vi "Create All Message Queues.vi"(8 "error in (no error)":cluster{"状态":bool, "代码":i32, "源":string} caption="错误输入（无错误）") -> (0 "error out":cluster{"状态":bool, "代码":i32, "源":string} caption="错误输出", 3 "消息队列输出":T1)   [LabVIEW 2014, in "Message Queue.lvlib"]
doc: "本VI用于创建应用程序所需的所有消息队列。如应用程序需要两个以上消息队列，可右键单击上面的“消息队列”常量并选择“打开自定义类型”，将新的消息队列添加至该自定义类型，然后通过本VI进行初始化。"
uses:
  Message Queue.lvlib
  All Message Queues.ctl
  Message Cluster.ctl
  Enqueue Message (Single).vi
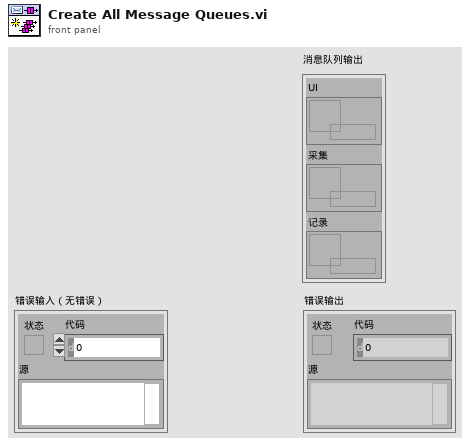
[diagram p1: front panel]
types:
  T1 = typedef "Message Queue.lvlib/All Message Queues.ctl" = cluster{"UI":refnum<queue>, "采集":refnum<queue>, "记录":refnum<queue>}
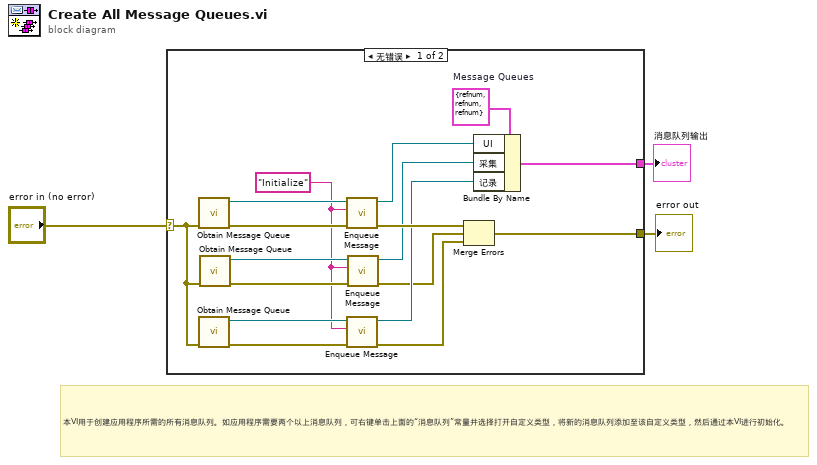
[diagram p0: block diagram]
diagram:
  # "本VI用于创建应用程序所需的所有消息队列。如应用程序需要两个以上消息队列，可右键单击上面的“消息队列”常量并选择打开自定义类型，将新的消息队列添加至该自定义类型，然后通过本VI进行初始化。"
  n1 = case shown="无错误" "error in (no error)" {
    selector: "error in (no error)" -> [w11 w21]
    tunnel: [w6 w21] -> w3
    tunnel: [w18 _] -> w2
    frame No Error {
      w10 = "Initialize" ("Message")
      w19 = T1 {"UI"=refnum, "采集"=refnum, "记录"=refnum}  # Message Queues
      n2 = call "Obtain Message Queue.vi"("error in (no error)"=w11) -> ("error out"=w17:cluster{"状态":bool, "代码":i32, "源":string}, "消息队列"=w16:refnum<queue>)  [unwired: 9 in]
      n3 = call "Obtain Message Queue.vi"("error in (no error)"=w11) -> ("error out"=w13:cluster{"状态":bool, "代码":i32, "源":string}, "消息队列"=w12:refnum<queue>)  [unwired: 9 in]
      n4 = call "Obtain Message Queue.vi"("error in (no error)"=w11) -> ("error out"=w14:cluster{"状态":bool, "代码":i32, "源":string}, "消息队列"=w15:refnum<queue>)  [unwired: 9 in]
      n5 = call-poly "Enqueue Message.vi"("error in (no error)"=w17, "消息"=w10, "消息队列"=w16) -> ("error out"=w20:cluster{"状态":bool, "代码":i32, "源":string}, "消息队列副本"=w9:refnum<queue>)  [unwired: 7 in]
      n6 = call-poly "Enqueue Message.vi"("error in (no error)"=w13, "消息"=w10, "消息队列"=w12) -> ("error out"=w4:cluster{"状态":bool, "代码":i32, "源":string}, "消息队列副本"=w7:refnum<queue>)  [unwired: 7 in]
      n7 = call-poly "Enqueue Message.vi"("error in (no error)"=w14, "消息"=w10, "消息队列"=w15) -> ("error out"=w5:cluster{"状态":bool, "代码":i32, "源":string}, "消息队列副本"=w8:refnum<queue>)  [unwired: 7 in]
      n8 = Merge Errors(w20, w5, w4) -> (w6:errorcluster)
      n9 = Bundle By Name(cluster=w19, "UI"=w9, "采集"=w8, "记录"=w7) -> (w18:T1)
    }
    frame Error {
    }
  }
  "消息队列输出" <- w2
  "error out" <- w3
